vi "Cleanup.vi"(8 "error in (no error)":errorcluster, 11 "Device in":refnum<class "Device.lvclass">) -> (0 "error out":errorcluster)   [LabVIEW 2020, in "PicoG-App.lvlib" / "Device.lvclass"]
uses:
  Device.lvclass
  Device.lvclass/Device.ctl
  Builds/picoG/ppl/PicoG-Core.lvlibp/PicoG-Processor/PicoG-Core/Resource/Resource.lvclass
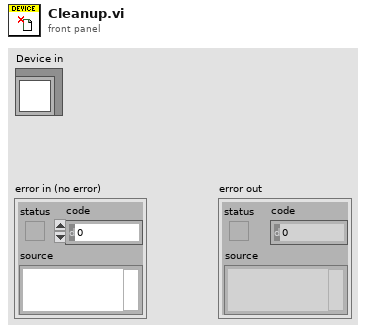
[diagram p1: front panel]
types:
  T1 = typedef "PicoG-App.lvlib/Device.lvclass/Resource Ref.ctl" = cluster{"Resource":refnum<class "Resource.lvclass">, "Open":bool, "At Prompt":bool, "Running":bool}
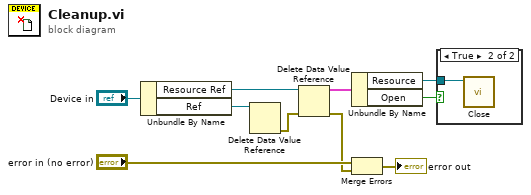
[diagram p0: block diagram]
diagram:
  n1 = Unbundle By Name("Device in") -> ("Resource Ref"=w7:refnum<data-value>, "Ref"=w8:refnum<data-value>)
  n2 = Delete Data Value Reference(data value reference=w8) -> (error out=w6:errorcluster)  [unwired: 1 in, 1 out]
  n3 = Delete Data Value Reference(data value reference=w7, error in=w6) -> (data value=w3:T1, error out=w4:errorcluster)
  n4 = Unbundle By Name(w3) -> ("Resource"=w1:refnum<class "Resource.lvclass">, "Open"=w2:bool)
  n5 = Merge Errors("error in (no error)", w4) -> (→"error out":errorcluster)
  n6 = case shown="True" w2 {
    tunnel: w1 -> [_ w11]
    frame False {
    }
    frame True {
      n7 = call-dynamic "Close.vi"("DeployResource in"=w11) -> ()  [unwired: 9 in, 2 out]
    }
  }
